vi "Read Expression.vi"(8 "error in (no error)":errorcluster, 11 "Cron in":refnum<class "Cron.lvclass">) -> (0 "error out":errorcluster, 2 "Expression":string, 3 "Cron out":refnum<class "Cron.lvclass">)   [LabVIEW 2013, in "openCron.lvlib" / "Cron.lvclass"]
uses:
  Cron.lvclass
  Cron.lvclass/Cron.ctl
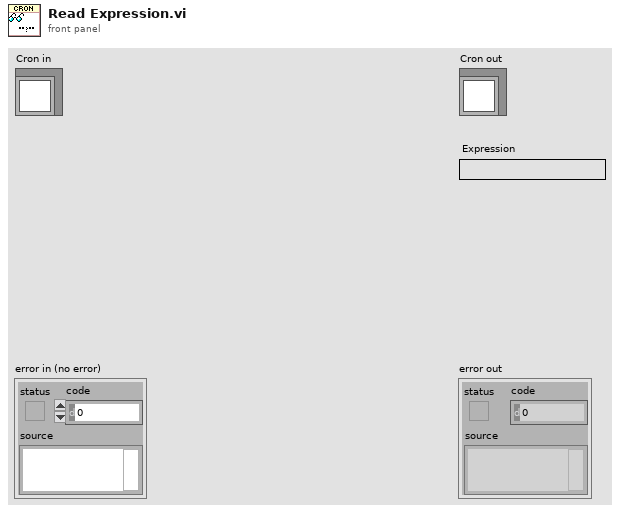
[diagram p1: front panel]
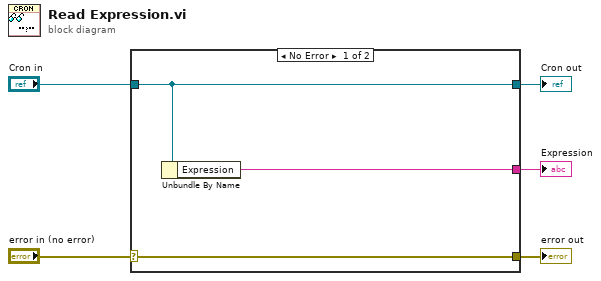
[diagram p0: block diagram]
diagram:
  n1 = case shown="No Error" "error in (no error)" {
    selector: "error in (no error)" -> [w8 w9]
    tunnel: [w8 w9] -> w4
    tunnel: [w7 w10] -> w2
    tunnel: "Cron in" -> [w7 w10]
    tunnel: [w6 _] -> w1
    frame No Error {
      n2 = Unbundle By Name(w7) -> ("Expression"=w6:string)
    }
    frame Error {
    }
  }
  "error out" <- w4
  "Cron out" <- w2
  "Expression" <- w1
